vi "subUpdateCSharpProjectFile.vi"(8 "error in (no error)":errorcluster, 11 ".csproj path":path) -> (0 "error out":errorcluster, 3 ".csproj path out":path)   [LabVIEW 2015, in "veristand-steps-build-tools.lvlib"]
uses:
  veristand-steps-build-tools.lvlib
  <vilib>/xml/Load XML File.vi
  <vilib>/xml/Close Reference(Node).vi
  <vilib>/xml/Close Reference(NNMap).vi
  <userlib>/Simple XML/_polymorphics/Create Tag - Child with Text.vi
  <vilib>/xml/NI_XML.lvlib
  <resource>/objmgr/DOMUserDefRef.rc
  <userlib>/Simple XML/Simple XML.lvlib
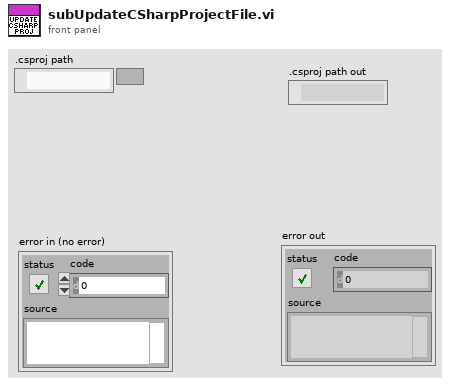
[diagram p1: front panel]
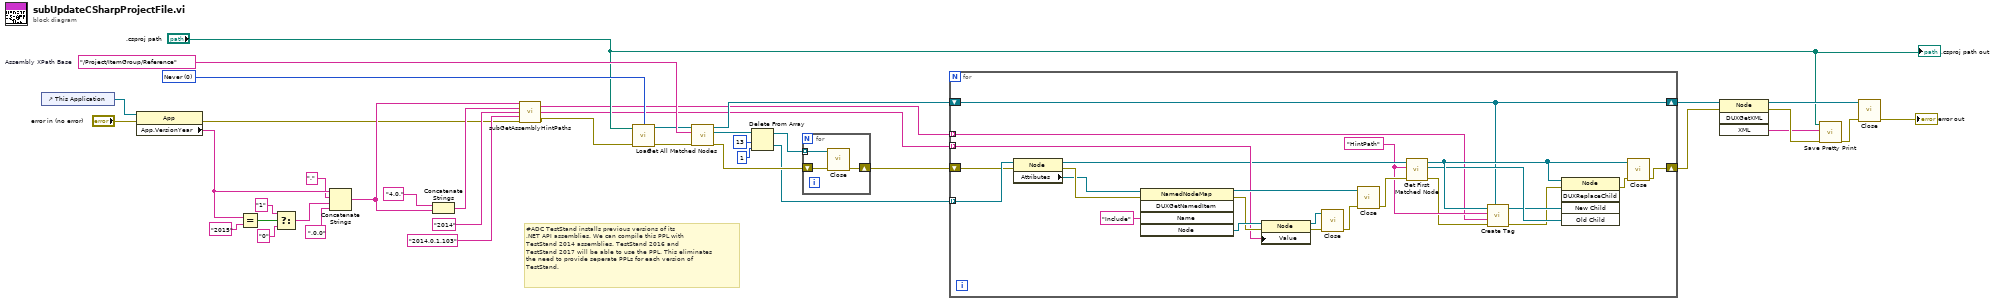
[diagram p0: block diagram]
diagram:
  w25 = "/Project/ItemGroup/Reference"  # Assembly XPath Base
  w22 = 0 items=["Never", "Always", "Auto"] ("validate on load (Auto)")
  # "#ADC TestStand installs previous versions of its \n.NET API assemblies. We can compile this PPL with\nTestStand 2014 assemblies. TestStand 2016 and\nTestStand 2017 will be able to use the PPL. This eliminates\nthe need to provide seperate PPLs for each version of\nTestStand."
  n1 = control-ref of="This Application"() -> (w17:refnum<vi>)
  n2 = property class="App"(reference=w17, error in="error in (no error)") -> (error out=w3:errorcluster, "App.VersionYear"=w14:string)  [unwired: 1 out]
  n3 = Equal?(x=w14, y="2015") -> (x = y?=w12:bool)
  n4 = Select(t="1" ("string"), s=w12, f="0" ("string")) -> (s? t:f=w9:string)
  n5 = Concatenate Strings(w14, "." ("string"), w9, ".0.0" ("string")) -> (w6:string)
  n6 = Concatenate Strings("4.0." ("string"), w6) -> (w4:string)
  n7 = call "subGetAssemblyHintPaths.vi"("VeriStand assembly version string (2014.0.0.0)"=w6, "VeriStand GAC assembly version (4.0.2014.0.0.0)"=w4, "TestStand version string (2014)"="2014", "TestStand assembly version (2014.0.0.0)"="2014.0.1.103", "error in"=w3) -> ("New Assembly Hint Paths"=w18:string[], "New Assembly Include Paths"=w19:string[], "error out"=w20:errorcluster)  [unwired: 8 in]
  n8 = call-poly <vilib>:"Load.vi"("path to XML document"=".csproj path", "validate on load (Auto)"=w22, "error in (no error)"=w20) -> ("DOM document out"=w24:refnum<k20>, "error out"=w23:errorcluster)  [unwired: 10 in, 1 out]
  n9 = call <vilib>:"Get All Matched Nodes.vi"("error in (no error)"=w23, "XPath expression"=w25, "node in"=w24) -> ("error out"=w31:errorcluster, "node result array"=w26:refnum<k20>[], "node out"=w38:refnum<k20>)  [unwired: 6 in]
  n10 = Delete From Array(array=w26, length=13, index=1 ("length")) -> (deleted portion=w29:refnum<k20>[], array with subset deleted=w30:refnum<k20>[])
  n11 = for {
    tunnel: w30 -> [w42] mode=indexing
    shift-right: [w40] -> w32
    shift-left: w31 -> [w41]
    n12 = call-poly <vilib>:"Close.vi"("error in (no error)"=w41, "node"=w42) -> ("error out"=w40:errorcluster)  [unwired: 7 in]
  }
  n13 = for {
    tunnel: w29 -> [w63] mode=indexing
    shift-right: [w57] -> w33
    shift-left: w32 -> [w62]
    tunnel: w19 -> [w56] mode=indexing
    tunnel: w18 -> [w44] mode=indexing
    shift-right: [w43] -> w39
    shift-left: w38 -> [w43]
    w51 = "HintPath" ("XPath expression")
    n14 = property class="Node"(reference=w63, error in=w62) -> (reference out=w52:refnum<k20>, error out=w66:errorcluster, "Attributes"=w64:refnum<k20>)
    n15 = invoke class="NamedNodeMap" method="DUXGetNamedItem"(reference=w64, error in=w66, "Name"="Include") -> (reference out=w58:refnum<k20>, error out=w60:errorcluster, "Node"=w61:refnum<k20>)  [unwired: 2 in, 2 out]
    n16 = property class="Node"(reference=w61, error in=w60, "Value"=w56) -> (reference out=w59:refnum<k20>, error out=w55:errorcluster)
    n17 = call-poly <vilib>:"Close.vi"("error in (no error)"=w55, "node"=w59) -> ("error out"=w54:errorcluster)  [unwired: 7 in]
    n18 = call-poly <vilib>:"Close.vi"("error in (no error)"=w54, "named node map"=w58) -> ("error out"=w53:errorcluster)  [unwired: 7 in]
    n19 = call <vilib>:"Get First Matched Node.vi"("error in (no error)"=w53, "XPath expression"=w51, "node in"=w52) -> ("error out"=w50:errorcluster, "node result"=w48:refnum<k20>, "node out"=w49:refnum<k20>)  [unwired: 6 in]
    n20 = call-poly <userlib>:"Create Tag.vi"("DOM document reference"=w43, "error in (no error)"=w50, "Text Data"=w44, "Tag Name"=w51, "Parent Element reference"=w49) -> ("error out"=w46:errorcluster, "Child Element reference"=w47:refnum<k20>)  [unwired: 5 in]
    n21 = invoke class="Node" method="DUXReplaceChild"(reference=w49, error in=w46, "New Child"=w47, "Old Child"=w48) -> (error out=w45:errorcluster)  [unwired: 1 in, 4 out]
    n22 = call-poly <vilib>:"Close.vi"("error in (no error)"=w45, "node"=w49) -> ("error out"=w57:errorcluster)  [unwired: 7 in]
  }
  n23 = invoke class="Node" method="DUXGetXML"(reference=w39, error in=w33) -> (reference out=w37:refnum<k20>, error out=w35:errorcluster, "XML"=w34:string)  [unwired: 2 in, 1 out]
  n24 = call <userlib>:"Save Pretty Print.vi"("error in (no error)"=w35, "Pretty XML String"=w34, "XML file path"=".csproj path") -> ("error out"=w36:errorcluster)  [unwired: 7 in, 1 out]
  n25 = call-poly <vilib>:"Close.vi"("error in (no error)"=w36, "node"=w37) -> ("error out"=→"error out":errorcluster)  [unwired: 7 in]
  ".csproj path out" <- ".csproj path"
